vi "SS Send Data.vi"(8 "error in (no error)":errorcluster, 9 "Values":dbl[](array[numeric]), 10 "Reading Names":string[](array[string]), 11 "Data Q":refnum<queue>) -> (0 "error out":errorcluster)   [LabVIEW 2021]
uses:
  SS cluster Data Queue type.ctl
  SS cluster Data Queue Data 1D Array.ctl
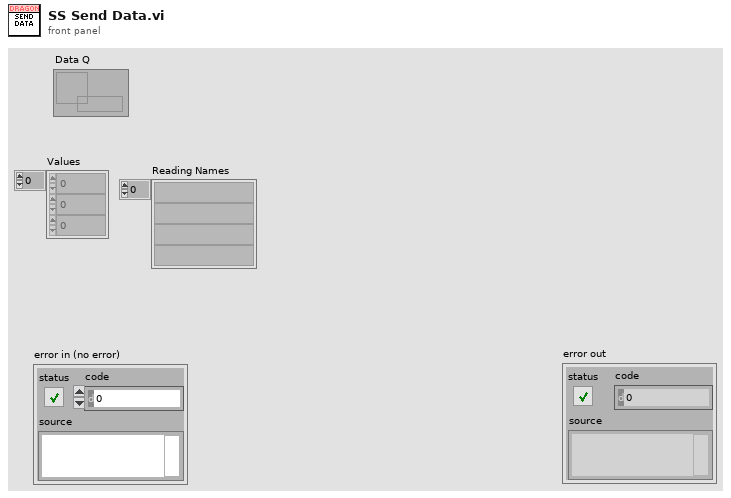
[diagram p1: front panel]
types:
  T1 = typedef "SS cluster Data Queue Data 1D Array.ctl" = cluster{"Reading Names":string[], "Values":dbl[]}
  T2 = typedef "SS cluster Data Queue type.ctl" = cluster{"Source":string, "Type":string, "Data":variant}
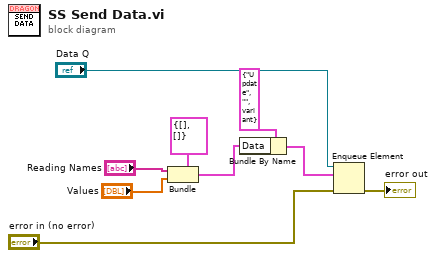
[diagram p0: block diagram]
diagram:
  n1 = Bundle(cluster=T1 {"Reading Names"=[], "Values"=[]} ("Data Q 1D Array"), "Reading Names"="Reading Names", "Values"="Values") -> (w2:T1)
  n2 = Bundle By Name(cluster=T2 {"Source"="Update", "Type"="", "Data"=variant} ("element"), "Data"=w2) -> (w1:T2)
  n3 = Enqueue Element(queue="Data Q", element=w1, error in (no error)="error in (no error)") -> (error out=→"error out":errorcluster)  [unwired: 1 in, 2 out]
